vi "StopAndClearAllCache.vi"(5 "error in (no error)":errorcluster) -> (19 "error out":errorcluster)   [LabVIEW 2018, in "LcWebView.lvclass"]
uses:
  LcWebView.lvclass
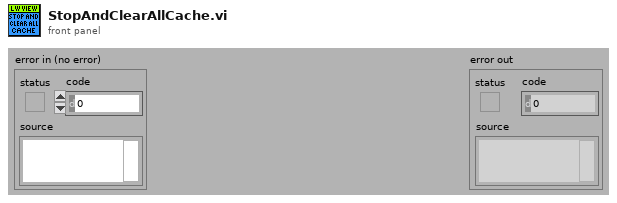
[diagram p1: front panel]
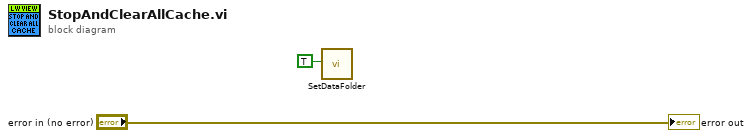
[diagram p0: block diagram]
diagram:
  n1 = call "SetDataFolder.vi"("JustKillAllSavedReferences(False)"=TRUE) -> ()  [unwired: 15 in, 4 out]
  "error out" <- "error in (no error)"
